vi "Event Structure - Generated Signal.vi"() -> ()   [LabVIEW 2011]
doc: "Use this template to build a user interface event handler design pattern. Use this pattern for dialog boxes and other user interfaces. You also can create and execute user-defined events that the VI can handle the same way as user interface events."
uses:
  <vilib>/Analysis/4window.llb/windowTd.ctl
  <vilib>/DAQmx/read.llb/DAQmx Read (Analog 1D Wfm NChan NSamp).vi
  <vilib>/DAQmx/create/channels.llb/DAQmx Create Channel (AI-Voltage-Basic).vi
  <vilib>/DAQmx/configure/timing.llb/DAQmx Timing (Sample Clock).vi
  <vilib>/DAQmx/miscellaneous.llb/DAQmx Fill In Error Info.vi
  <vilib>/measure/maspectr.llb/FFT Power Spectrum and PSD for N Chan.vi
  <vilib>/measure/NI_MAPro.lvlib
  <vilib>/Analysis/NI_AALPro.lvlib
panel:
  in  "Tab Control 2":enum32{"Time Domain Signal", "Frequency Domain"}(tab)
  out "Waveform Graph":waveform(dbl)[](graph)
  out "FFT Graph":cluster{"f0":dbl, "df":dbl, "magnitude":dbl[]}[](graph)
  in  "Analyze Data":bool
  in  "Generate Data":bool
  in  "Tab Control":T1(tab)
  in  "Pin 1":tag
  in  "Pin 2":tag
  in  "Noise Amplitude (mV)":dbl
  in  "Sample Per Channel":i32=240
  in  "Frequency (Hz)":dbl=2000.0 format="%0.2f"
  in  "Amplitude (V)":dbl=2.5
  in  "Generated Frequency (Hz)":dbl=50.0
  in  "dB On (F)":bool
  in  "window":T2=1 items=["Rectangle"=0, "Hanning"=1, "Hamming"=2, "Blackman-Harris"=3, "Exact Blackman"=4, "Blackman"=5, "Flat Top"=6, "4 Term B-Harris "=7, "7 Term B-Harris"=8, "Low Sidelobe"=9, "Blackman Nuttall"=11, "Triangle"=30, "Bartlett-Hanning"=31, "Bohman"=32, "Parzen"=33, "Welch"=34, "Kaiser"=60, "Dolph-Chebyshev"=61, "Gaussian"=62]
  out "Error":errorcluster
  in  "Take Data":bool
  in  "stop":bool
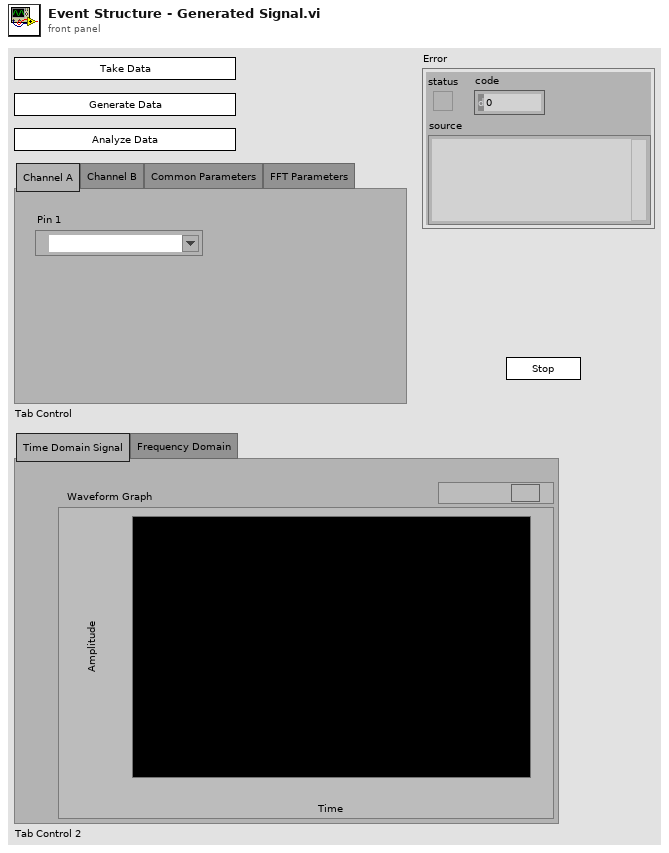
[diagram p1: front panel]
types:
  T1 = enum32{"Channel A", "Channel B", "Common Parameters", "FFT Parameters"}
  T2 = typedef "NI_AALPro.lvlib/windowTd.ctl" = u32
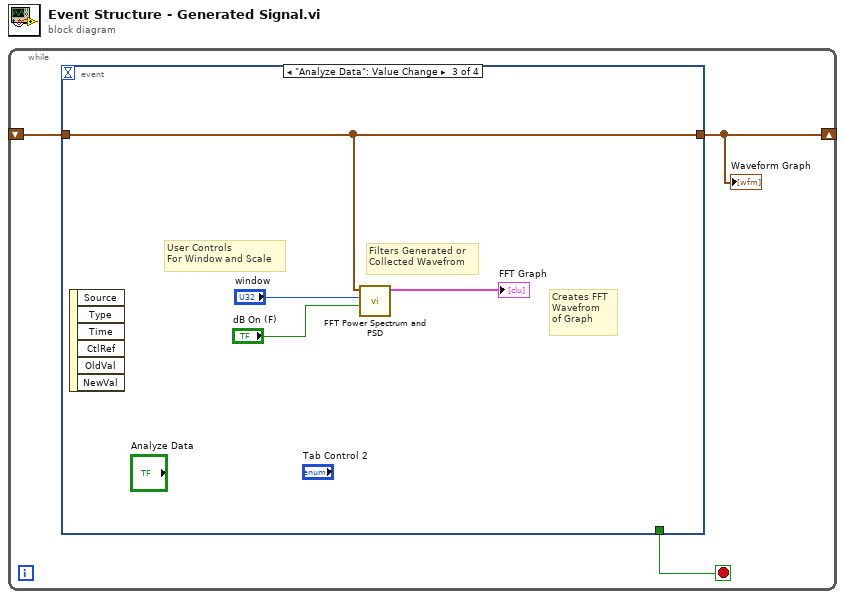
[diagram p0: block diagram]
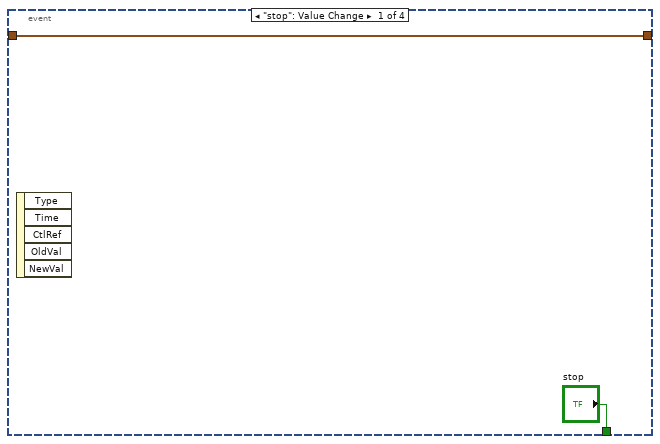
[diagram p2: hidden frame]
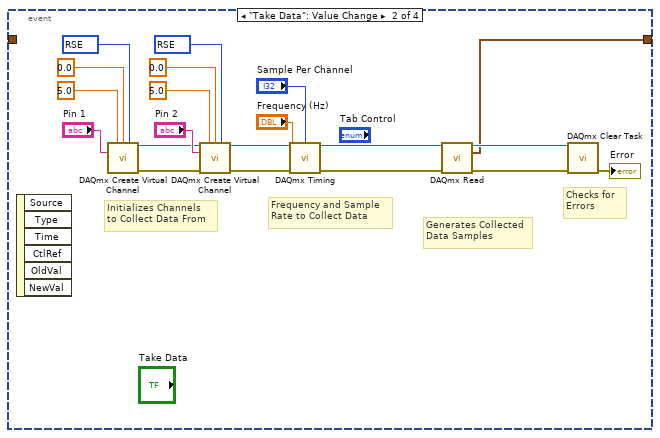
[diagram p3: hidden frame]
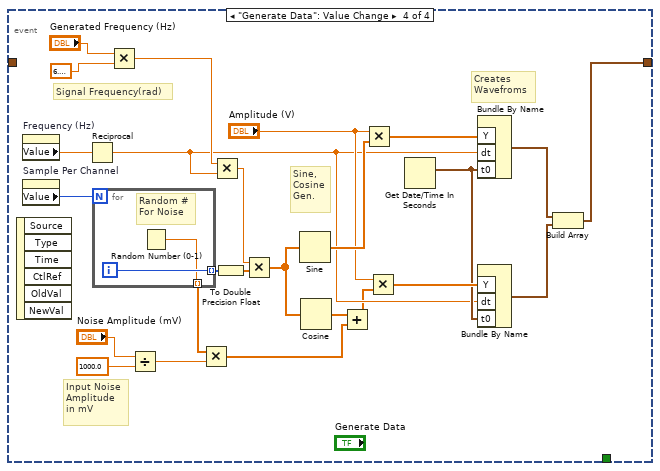
[diagram p4: hidden frame]
diagram:
  n1 = while {
    shift-right: [w1] -> _
    shift-left: _ -> [w2]
    stop <- w3 stop-if-true
    n2 = event shown="[2] \"Analyze Data\": Value Change" {
      selector: _ -> [_ _ _ _]
      dyn-events: _ -> [_ _ _ _]
      timeout: _ -> [_ _ _ _]
      tunnel: ["stop" _ _ _] -> w3
      tunnel: [w4 w6 w29 w44] -> w1
      tunnel: w2 -> [w4 _ w29 _]
      event "stop": Value Change {
        n3 = event-data() -> ()  [unwired: 1 in, 5 out]
      }
      event "Take Data": Value Change {
        w19 = 10083 items=["default"=-1, "RSE"=10083, "NRSE"=10078, "Differential"=10106, "Pseudodifferential"=12529] ("input terminal configuration")
        w23 = 10083 items=["default"=-1, "RSE"=10083, "NRSE"=10078, "Differential"=10106, "Pseudodifferential"=12529] ("input terminal configuration")
        # "Checks for \nErrors"
        # "Generates Collected\nData Samples"
        # "Frequency and Sample\nRate to Collect Data"
        # "Initializes Channels\nto Collect Data From"
        n4 = event-data() -> ()  [unwired: 1 in, 6 out]
        n5 = call-poly <vilib>:"DAQmx Create Virtual Channel.vi"("maximum value"=5.0, "minimum value"=0.0, "input terminal configuration"=w23, "physical channels"="Pin 1") -> ("task out"=w17:refnum<k21>, "error out"=w16:errorcluster)  [unwired: 10 in]
        n6 = call-poly <vilib>:"DAQmx Create Virtual Channel.vi"("task in"=w17, "maximum value"=5.0, "minimum value"=0.0, "input terminal configuration"=w19, "physical channels"="Pin 2", "error in"=w16) -> ("task out"=w12:refnum<k21>, "error out"=w10:errorcluster)  [unwired: 8 in]
        n7 = call-poly <vilib>:"DAQmx Timing.vi"("task/channels in"=w12, "samples per channel"="Sample Per Channel", "rate"="Frequency (Hz)", "error in"=w10) -> ("task out"=w11:refnum<k21>, "error out"=w9:errorcluster)  [unwired: 10 in]
        n8 = call-poly <vilib>:"DAQmx Read.vi"("task/channels in"=w11, "error in"=w9) -> ("task out"=w15:refnum<k21>, "data"=w6:waveform(dbl)[], "error out"=w14:errorcluster)  [unwired: 11 in]
        n9 = call <vilib>:"DAQmx Clear Task.vi"("task in"=w15, "error in"=w14) -> ("error out"=→"Error":errorcluster)  [unwired: 13 in]
      }
      event "Analyze Data": Value Change {
        # "Creates FFT \nWavefrom\nof Graph"
        # "Filters Generated or\nCollected Wavefrom"
        # "User Controls \nFor Window and Scale"
        n10 = event-data() -> ()  [unwired: 1 in, 6 out]
        n11 = call-poly <vilib>:"FFT Power Spectrum and PSD.vi"("dB On (F)"="dB On (F)", "window"="window", "time signals"=w29) -> ("Power Spectrum / PSD"=→"FFT Graph":cluster{"f0":dbl, "df":dbl, "magnitude":dbl[]}[])  [unwired: 5 in, 3 out]
      }
      event "Generate Data": Value Change {
        # "Creates \nWavefroms"
        # "Signal Frequency(rad)"
        # "Sine,\nCosine\nGen."
        # "Input Noise\nAmplitude\nin mV"
        n12 = event-data() -> ()  [unwired: 1 in, 6 out]
        n13 = property on="Frequency (Hz)" class="DigNum (strict)"() -> ("Value"=w38:dbl)  [unwired: 2 in, 2 out]
        n14 = property on="Sample Per Channel" class="DigNum (strict)"() -> ("Value"=w54:i32)  [unwired: 2 in, 2 out]
        n15 = Reciprocal(x=w38) -> (1/x=w40:dbl)
        n16 = for {
          N: w54 -> [_]
          tunnel: [w56] -> w53 mode=indexing
          tunnel: [w55] -> w34 mode=indexing
          i -> [w56]
          # "Random #\nFor Noise"
          n17 = Random Number (0-1)() -> (number: 0 to 1=w55:dbl)
        }
        n18 = Multiply(x="Generated Frequency (Hz)", y=6.283185307179586) -> (x*y=w41:dbl)
        n19 = Divide(x="Noise Amplitude (mV)", y=1000.0) -> (x/y=w35:dbl)
        n20 = Multiply(x=w34, y=w35) -> (x*y=w33:dbl[])
        n21 = Multiply(x=w41, y=w40) -> (x*y=w39:dbl)
        n22 = To Double Precision Float(number=w53) -> (double precision float=w52:dbl[])
        n23 = Multiply(x=w39, y=w52) -> (x*y=w32:dbl[])
        n24 = Sine(x=w32) -> (sin(x)=w51:dbl[])
        n25 = Cosine(x=w32) -> (cos(x)=w30:dbl[])
        n26 = Add(x=w30, y=w33) -> (x+y=w31:dbl[])
        n27 = Multiply(x="Amplitude (V)", y=w51) -> (x*y=w50:dbl[])
        n28 = Multiply(x="Amplitude (V)", y=w31) -> (x*y=w48:dbl[])
        n29 = Get Date/Time In Seconds() -> (seconds since 1Jan1904=w47:timestamp)
        n30 = Bundle By Name("Y"=w50, "dt"=w40, "t0"=w47) -> (w46:waveform(dbl))  [unwired: 1 in]
        n31 = Bundle By Name("Y"=w48, "dt"=w40, "t0"=w47) -> (w45:waveform(dbl))  [unwired: 1 in]
        n32 = Build Array(w46, w45) -> (w44:waveform(dbl)[])
      }
    }
    "Waveform Graph" <- w1
  }
